vi "BLEwrite_from_file.vi"() -> ()   [LabVIEW 2014]
uses:
  <vilib>/BLE/type_def/address_type.ctl
  <vilib>/BLE/type_def/connection_status_bundle.ctl
panel:
  in  "Control":enum32{"Control Disk", "Diskview from File"}(tab)
  in  "?":bool
  in  "?":bool
  in  "?":bool
  in  "?":bool
  in  "?":bool
  in  "?":bool
  in  "?":bool
  in  "?":bool
  in  "?":bool
  in  "?":bool
  in  "?":bool
  in  "?":bool
  in  "?":bool
  in  "?":bool
  in  "?":bool
  in  "?":bool
  in  "?":bool
  in  "?":bool
  in  "?":bool
  in  "?":bool
  in  "?":bool
  in  "?":bool
  in  "?":bool
  in  "?":bool
  in  "?":bool
  in  "?":bool
  in  "?":bool
  in  "?":bool
  in  "?":bool
  in  "?":bool
  in  "?":bool
  in  "?":bool
  in  "?":bool
  in  "?":bool
  in  "?":bool
  in  "?":bool
  in  "?":bool
  in  "?":bool
  in  "?":bool
  in  "?":bool
  in  "?":bool
  in  "?":bool
  in  "?":bool
  in  "?":bool
  in  "?":bool
  in  "?":bool
  in  "?":bool
  in  "?":bool
  in  "?":bool
  in  "?":bool
  in  "?":bool
  in  "?":bool
  in  "?":bool
  in  "?":bool
  in  "?":bool
  in  "?":bool
  in  "?":bool
  in  "?":bool
  in  "?":bool
  in  "?":bool
  in  "?":bool
  in  "?":bool
  in  "?":bool
  in  "?":bool
  in  "?":bool
  in  "?":bool
  in  "?":bool
  in  "?":bool
  in  "?":bool
  in  "?":bool
  in  "?":bool
  in  "?":bool
  in  "?":bool
  in  "?":bool
  in  "?":bool
  in  "?":bool
  in  "?":bool
  in  "?":bool
  in  "?":bool
  in  "?":bool
  in  "?":bool
  in  "?":bool
  in  "?":bool
  in  "?":bool
  in  "?":bool
  in  "?":bool
  in  "?":bool
  in  "?":bool
  in  "?":bool
  in  "?":bool
  in  "?":bool
  in  "?":bool
  in  "?":bool
  in  "?":bool
  in  "?":bool
  in  "?":bool
  in  "?":bool
  in  "?":bool
  in  "?":bool
  in  "?":bool
  in  "?":bool
  in  "?":bool
  in  "?":bool
  in  "?":bool
  in  "?":bool
  in  "?":bool
  in  "?":bool
  in  "?":bool
  in  "?":bool
  in  "?":bool
  in  "?":bool
  in  "?":bool
  in  "?":bool
  in  "?":bool
  in  "?":bool
  in  "?":bool
  in  "?":bool
  in  "?":bool
  in  "?":bool
  in  "?":bool
  in  "?":bool
  in  "?":bool
  in  "?":bool
  in  "?":bool
  in  "?":bool
  in  "?":bool
  in  "?":bool
  in  "?":bool
  out "Data sent":u8[](array[numeric]) format="%x"
  out "Expander":string
  out "Valve":string
  out "Write to device":bool
  out "Write from file":bool
  out "text":string[](array[string])
  out "Data sent 2":u8[](array[numeric]) format="%x"
  in  "file (use dialog)":path
  out "Expander 2":string
  out "Valve 2":string
  out "element":string
  out "Number of strings":i32
  out "?":bool
  out "?":bool
  out "?":bool
  out "?":bool
  out "?":bool
  out "?":bool
  out "?":bool
  out "?":bool
  out "?":bool
  out "?":bool
  out "?":bool
  out "?":bool
  out "?":bool
  out "?":bool
  out "?":bool
  out "?":bool
  out "?":bool
  out "?":bool
  out "?":bool
  out "?":bool
  out "?":bool
  out "?":bool
  out "?":bool
  out "?":bool
  out "?":bool
  out "?":bool
  out "?":bool
  out "?":bool
  out "?":bool
  out "?":bool
  out "?":bool
  out "?":bool
  out "?":bool
  out "?":bool
  out "?":bool
  out "?":bool
  out "?":bool
  out "?":bool
  out "?":bool
  out "?":bool
  out "?":bool
  out "?":bool
  out "?":bool
  out "?":bool
  out "?":bool
  out "?":bool
  out "?":bool
  out "?":bool
  out "?":bool
  out "?":bool
  out "?":bool
  out "?":bool
  out "?":bool
  out "?":bool
  out "?":bool
  out "?":bool
  out "?":bool
  out "?":bool
  out "?":bool
  out "?":bool
  out "?":bool
  out "?":bool
  out "?":bool
  out "?":bool
  out "?":bool
  out "?":bool
  out "?":bool
  out "?":bool
  out "?":bool
  out "?":bool
  out "?":bool
  out "?":bool
  out "?":bool
  out "?":bool
  out "?":bool
  out "?":bool
  out "?":bool
  out "?":bool
  out "?":bool
  out "?":bool
  out "?":bool
  out "?":bool
  out "?":bool
  out "?":bool
  out "?":bool
  out "?":bool
  out "?":bool
  out "?":bool
  out "?":bool
  out "?":bool
  out "?":bool
  out "?":bool
  out "?":bool
  out "?":bool
  out "?":bool
  out "?":bool
  out "?":bool
  out "?":bool
  out "?":bool
  out "?":bool
  out "?":bool
  out "?":bool
  out "?":bool
  out "?":bool
  out "?":bool
  out "?":bool
  out "?":bool
  out "?":bool
  out "?":bool
  out "?":bool
  out "?":bool
  out "?":bool
  out "?":bool
  out "?":bool
  out "?":bool
  out "?":bool
  out "?":bool
  out "?":bool
  out "?":bool
  out "?":bool
  out "?":bool
  out "?":bool
  out "?":bool
  out "?":bool
  out "?":bool
  out "?":bool
  out "?":bool
  out "?":bool
  in  "Mode Control":bool
  out "Expander Array":bool[](array[boolean])
  out "Expander number":u32
  in  "stop":bool
  out "Discover handles":bool
  out "Handle table":string[][](array[string])
  out "Disconnect":bool
  out "Connection Status":T1={"MAC Address"="", "cnx handle"=0, "cnx flags"=0, "Address Type"=125, "Connection Interval (ms)"=125, "Timeout(ms)"=125, "Latency"=0, "bonding handle"=0} {"Address Type" items=["Public", "Random"]}
  out "Connect to device":bool
  in  "Address Type":T2=1 items=["Public", "Random"]
  in  "MAC Address":string
  in  "COM Bluegiga in":refnum<visa-resource-name>="COM13"
  out "BLED112 Dongle Info":string
  # "Mac Adress: 7C:EC:79:69:6D:AE"
  # "Disk View"
  # "From file"
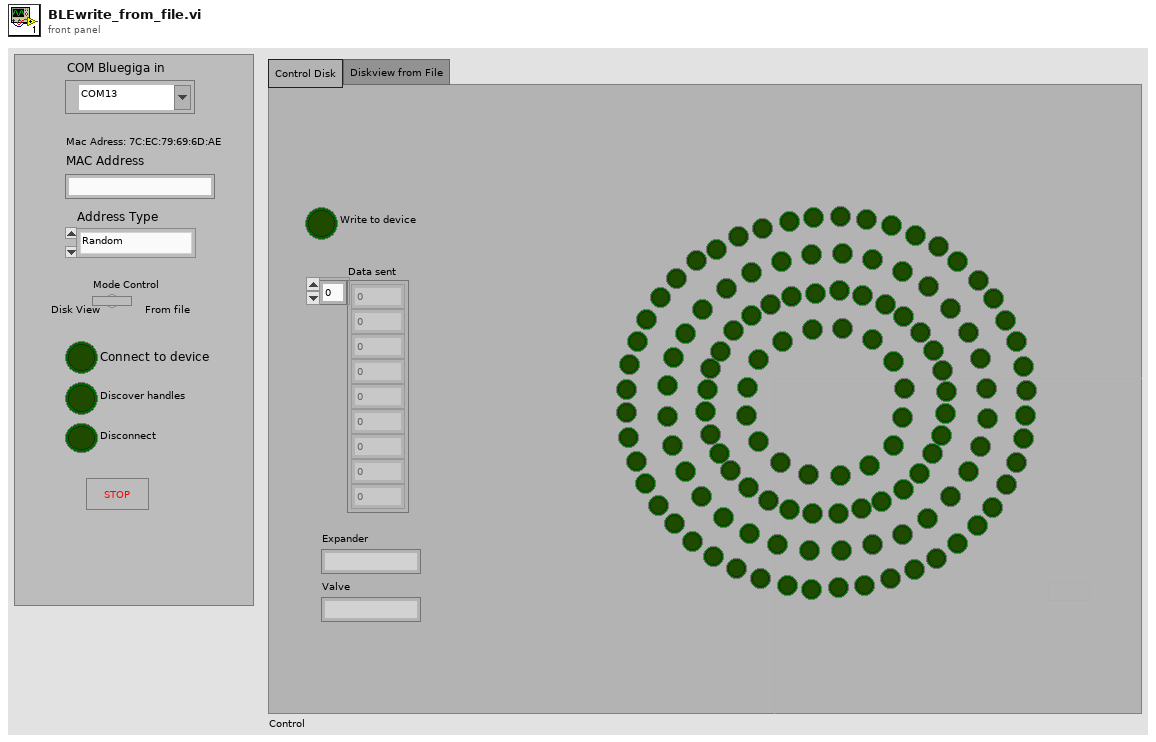
[diagram p1: front panel]
types:
  T1 = typedef "connection_status_bundle.ctl" = cluster{"MAC Address":string, "cnx handle":u8, "cnx flags":u8, "Address Type":T2, "Connection Interval (ms)":u16, "Timeout(ms)":u16, "Latency":u16, "bonding handle":u8}
  T2 = typedef "address_type.ctl" = u8
  T3 = cluster{"[0]":bool, "[1]":bool, "[2]":bool, "[3]":bool, "[4]":bool, "[5]":bool, "[6]":bool, "[7]":bool, "[8]":bool}
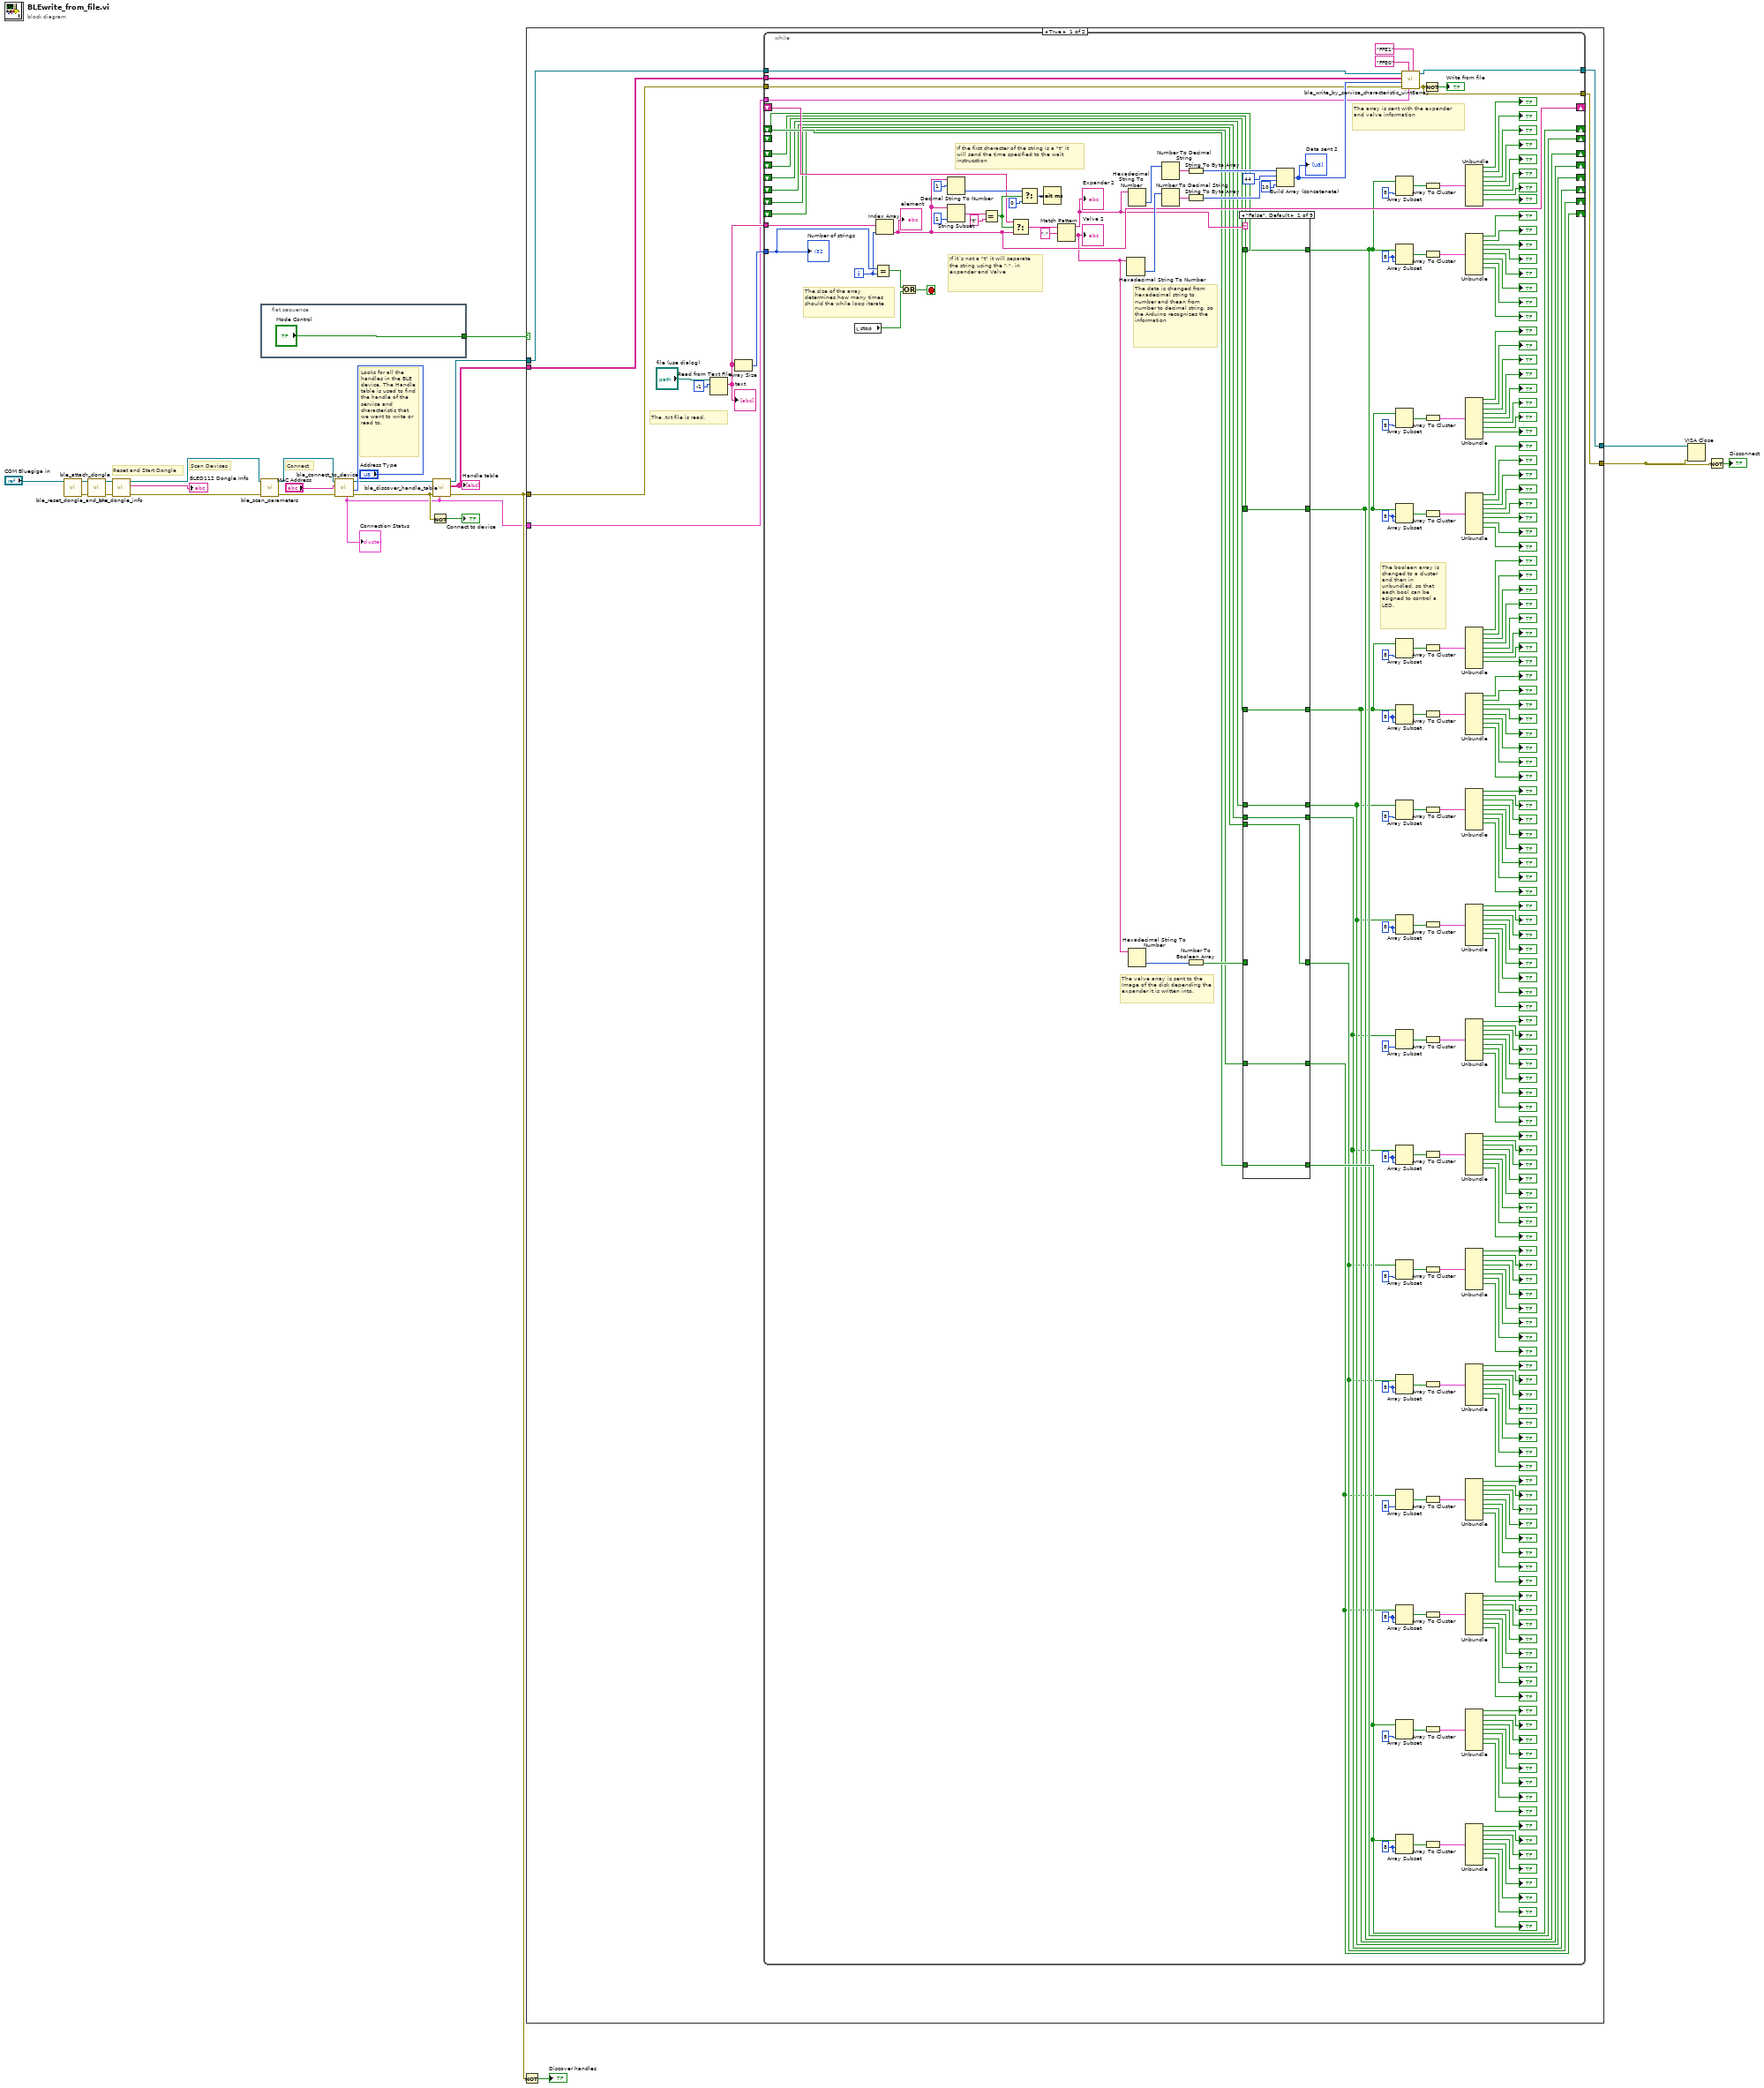
[diagram p0: block diagram]
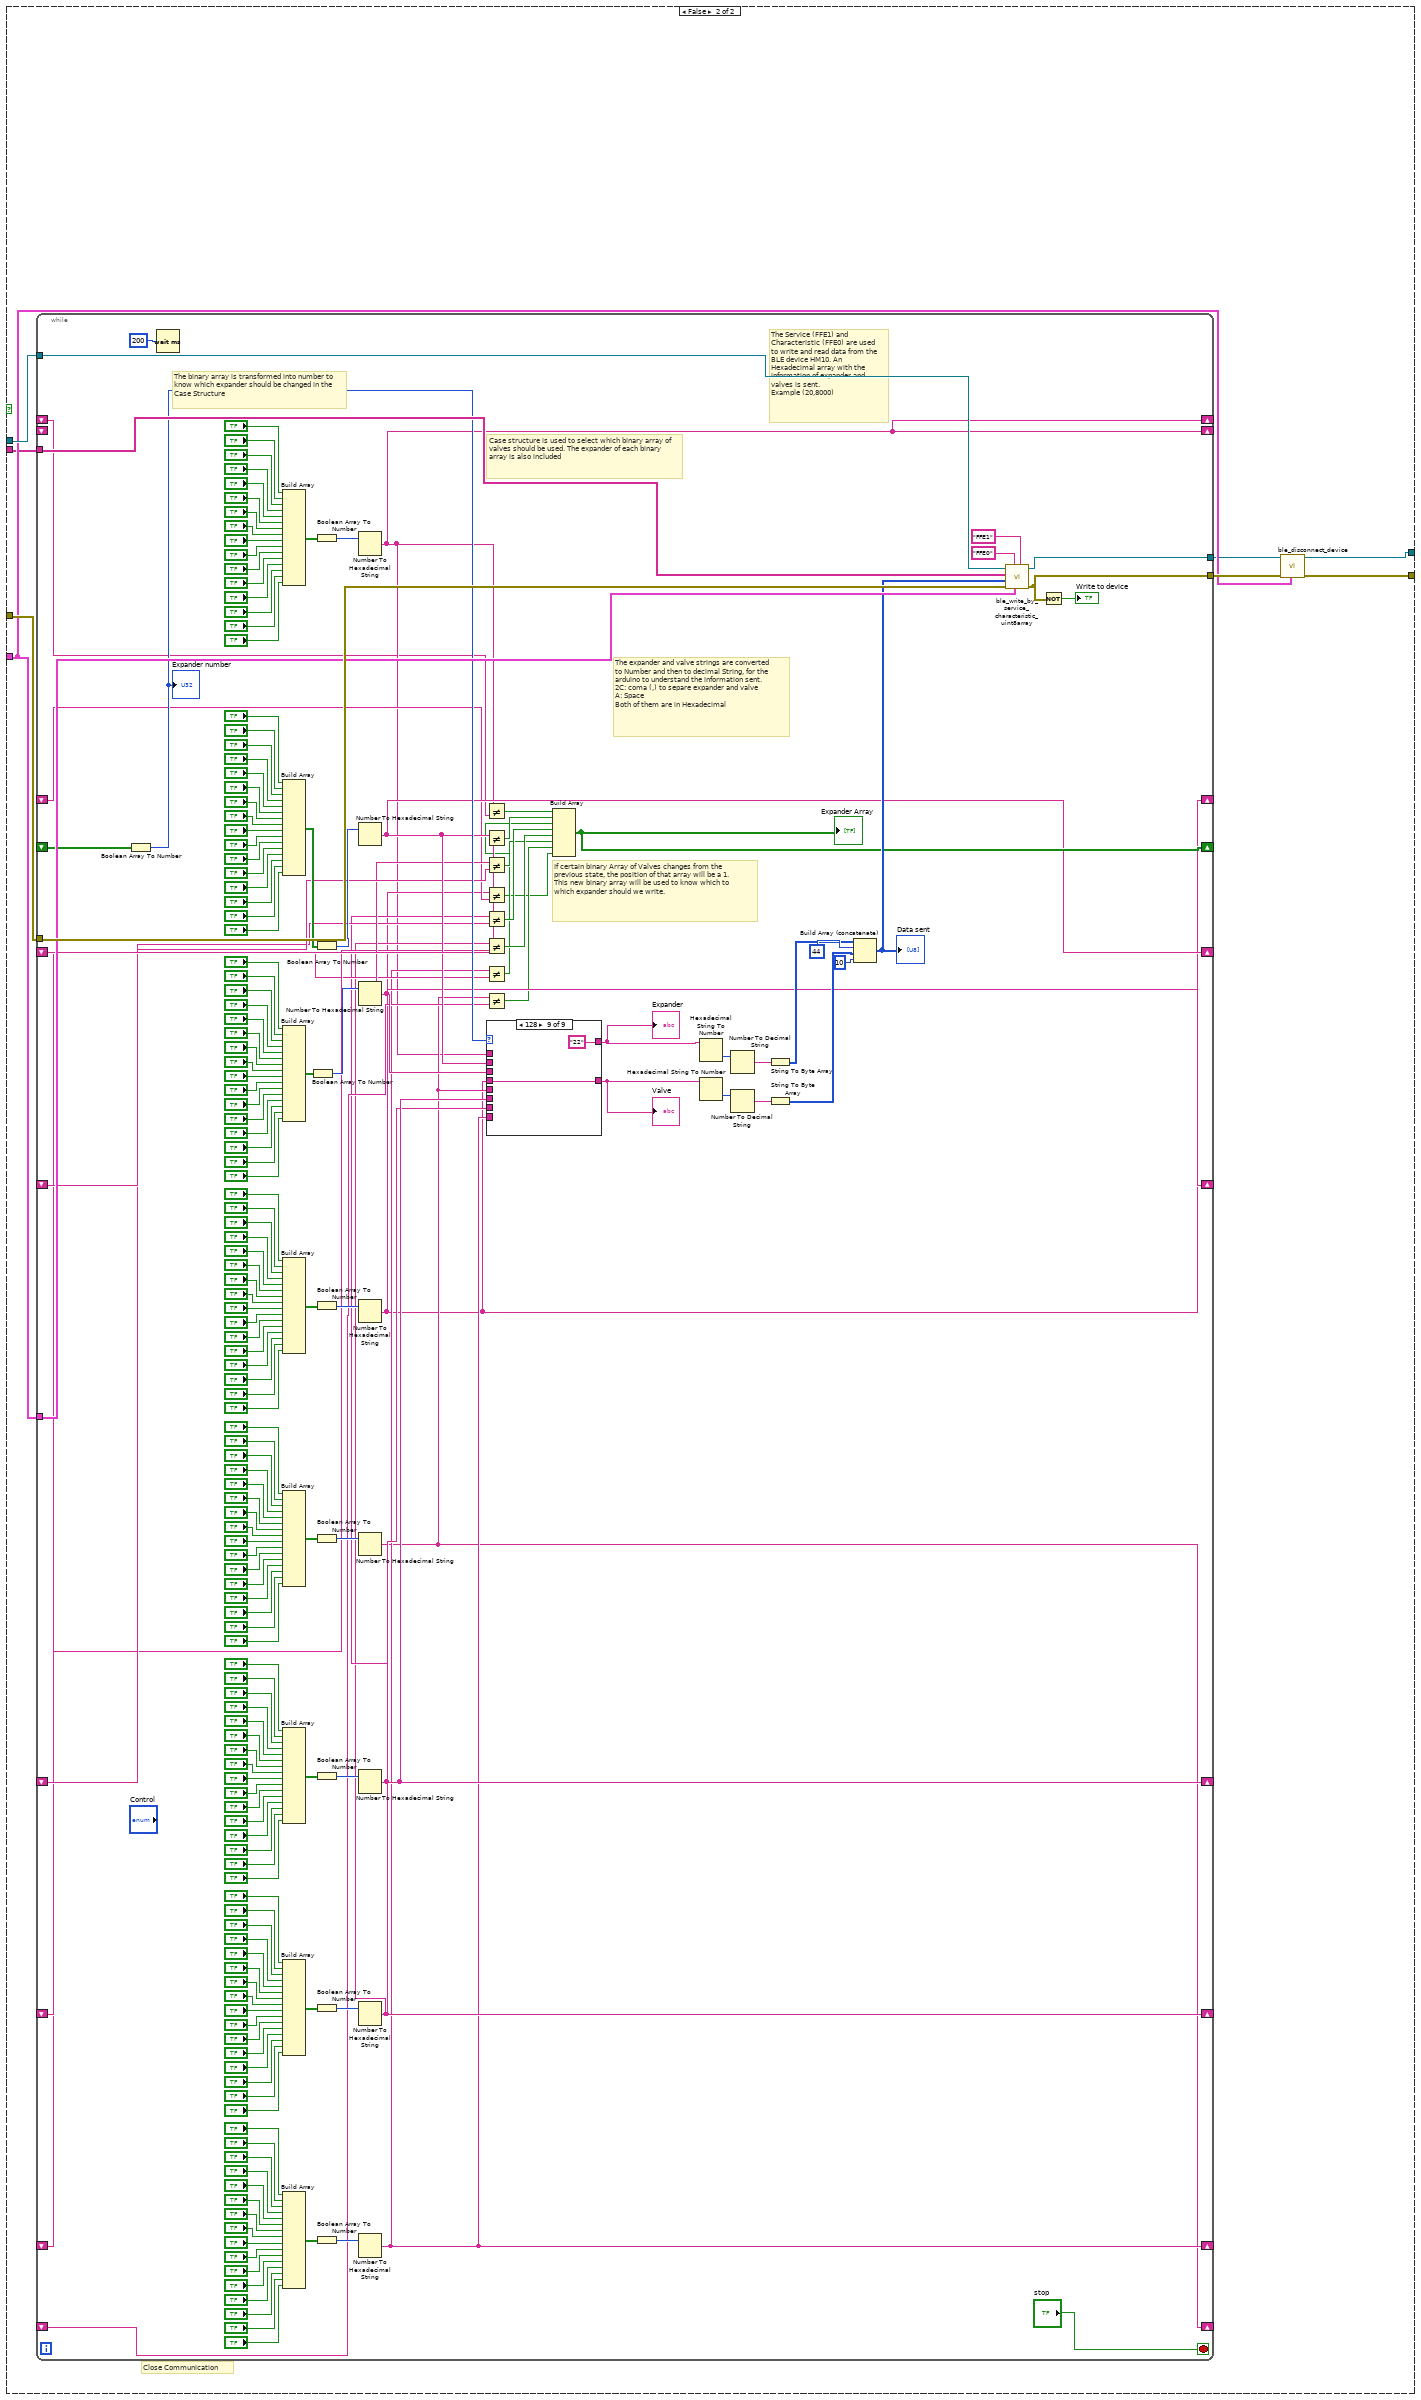
[diagram p10: hidden frame]
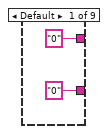
[diagram p11: hidden frame]
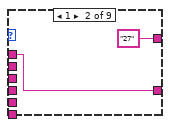
[diagram p12: hidden frame]
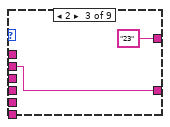
[diagram p13: hidden frame]
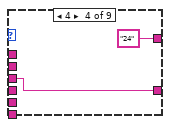
[diagram p14: hidden frame]
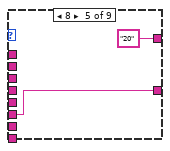
[diagram p15: hidden frame]
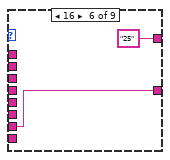
[diagram p16: hidden frame]
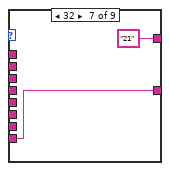
[diagram p17: hidden frame]
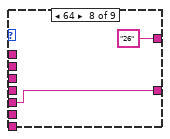
[diagram p18: hidden frame]
diagram:
  # "Reset and Start Dongle"
  # "Scan Devices"
  # "Connect"
  # "Looks for all the handles in the BLE device. The Handle table is used to find the handle of the service and characteristic that we want to write or read to."
  n1 = call <vilib>:"ble_reset_dongle_and_cnx.vi"("COM Bluegiga in"="COM Bluegiga in") -> ("error out"=w19:errorcluster, "COM Bluegiga out"=w17:refnum<visa-resource-name>)  [unwired: 9 in]
  n2 = call <vilib>:"ble_attach_dongle.vi"("error in (no error)"=w19, "COM Bluegiga in"=w17) -> ("error out"=w21:errorcluster, "COM Bluegiga out"=w20:refnum<visa-resource-name>)  [unwired: 8 in]
  n3 = call <vilib>:"ble_dongle_info.vi"("error in (no error)"=w21, "COM Bluegiga in"=w20) -> ("error out"=w22:errorcluster, "info"=→"BLED112 Dongle Info":string, "COM Bluegiga out"=w23:refnum<visa-resource-name>)  [unwired: 7 in]
  n4 = flat-sequence {
    tunnel: ["Mode Control"] -> w1
    frame #0 {
    }
  }
  n5 = call <vilib>:"ble_scan_parameters.vi"("error in (no error)"=w22, "COM Bluegiga in"=w23) -> ("error out"=w13:errorcluster, "COM Bluegiga out"=w14:refnum<visa-resource-name>)  [unwired: 7 in, 1 out]
  n6 = call <vilib>:"ble_connect_to_device.vi"("Address Type"="Address Type", "error in (no error)"=w13, "MAC Address"="MAC Address", "COM Bluegiga in"=w14) -> ("error out"=w7:errorcluster, "COM Bluegiga out"=w8:refnum<visa-resource-name>, "Connection Status"=w3:T1)  [unwired: 5 in]
  "Connection Status" <- w3
  n7 = Not(x=w7) -> (.not. x?=→"Connect to device":bool)
  n8 = call <vilib>:"ble_discover_handle_table.vi"("Connection Status"=w3, "error in (no error)"=w7, "COM Bluegiga in"=w8) -> ("error out"=w4:errorcluster, "Handle table"=w2:string[][], "COM Bluegiga out"=w5:refnum<visa-resource-name>)  [unwired: 6 in]
  "Handle table" <- w2
  n9 = Not(x=w4) -> (.not. x?=→"Discover handles":bool)
  n10 = case shown="True" w1 {
    tunnel: [w27 w347] -> w11
    tunnel: [w26 w346] -> w9
    tunnel: w5 -> [w30 w345]
    tunnel: w4 -> [w29 w344]
    tunnel: w3 -> [w28 w342]
    tunnel: w2 -> [w31 w341]
    frame True {
      # "The .txt file is read."
      n11 = Read from Text File(file (use dialog)="file (use dialog)", count=-1) -> (text=w32:string[])  [unwired: 2 in, 3 out]
      "text" <- w32
      n12 = Array Size(array=w32) -> (size(s)=w33:i32)
      n13 = while {
        tunnel: w33 -> [w267]
        tunnel: w32 -> [w253]
        tunnel: w31 -> [w251]
        tunnel: w30 -> [w250]
        tunnel: w29 -> [w249]
        tunnel: w28 -> [w248]
        tunnel: [w247] -> w27
        tunnel: [w246] -> w26
        shift-right: [w213] -> _
        shift-left: _ -> [w214]
        shift-right: [w54] -> _
        shift-left: _ -> [w53]
        shift-right: [w52] -> _
        shift-left: _ -> [w51]
        shift-right: [w50] -> _
        shift-left: _ -> [w49]
        shift-right: [w48] -> _
        shift-left: _ -> [w47]
        shift-right: [w46] -> _
        shift-left: _ -> [w45]
        shift-right: [w44] -> _
        shift-left: _ -> [w43]
        shift-right: [w42] -> _
        shift-left: _ -> [w41]
        shift-right: [w40] -> _
        shift-left: _ -> [w39]
        i -> [w254]
        stop <- w36 stop-if-true
        w170 = 8 ("length 2")
        w176 = 8 ("length 2")
        w182 = 8 ("length 2")
        w188 = 8 ("length 2")
        w194 = 8 ("length 2")
        w200 = 8 ("length 2")
        w206 = 8 ("length 2")
        w233 = 8 ("length 2")
        # "The boolean array is changed to a cluster and then in unbundled, so that each bool can be asigned to control a LED."
        # "The valve array is sent to the Image of the disk depending the expander it is written into."
        # "The data is changed from hexadecimal string to number and thean from number to decimal string, so the Arduino recognizes the information"
        # "The array is sent with the expander and valve information"
        # "If it´s not a \"t\" it will separate the string using the \",\", in expander and Valve"
        # "If the first character of the string is a \"t\" it will send the time specified to the wait instrucction"
        # "The size of the array determines how many times should the while loop iterate"
        n14 = local read "stop"() -> (w37:bool)
        n15 = Equal?(x=w267, y=w254) -> (x = y?=w38:bool)
        n16 = Index Array(array=w253, index=w254) -> (element=w213:string)
        "element" <- w213
        n17 = Or(x=w38, y=w37) -> (x .or. y?=w36:bool)
        n18 = Decimal String To Number(string=w213, offset=1 ("offset (0)")) -> (number=w240:i32)  [unwired: 1 in, 1 out]
        n19 = String Subset(string=w213, length (rest)=1 ("length (rest)")) -> (substring=w244:string)  [unwired: 1 in]
        n20 = Equal?(x=w244, y="t") -> (x = y?=w241:bool)
        n21 = Select(t=w214, s=w241, f=w213) -> (s? t:f=w242:string)
        n22 = Select(t=w240, s=w241, f=0) -> (s? t:f=w239:i32)
        n23 = Wait (ms)(milliseconds to wait=w239) -> ()  [unwired: 1 out]
        n24 = Match Pattern(string=w242, regular expression=",") -> (before substring=w210:string, after substring=w212:string)  [unwired: 1 in, 2 out]
        "Expander 2" <- w210
        "Valve 2" <- w212
        n25 = Hexadecimal String To Number(string=w212) -> (number=w260:u32)  [unwired: 2 in, 1 out]
        n26 = Hexadecimal String To Number(string=w210) -> (number=w263:u32)  [unwired: 2 in, 1 out]
        n27 = Hexadecimal String To Number(string=w212) -> (number=w211:u32)  [unwired: 2 in, 1 out]
        n28 = Number To Decimal String(number=w263) -> (decimal integer string=w262:string)  [unwired: 1 in]
        n29 = Number To Decimal String(number=w260) -> (decimal integer string=w259:string)  [unwired: 1 in]
        n30 = String To Byte Array(string=w262) -> (unsigned byte array=w257:u8[])
        n31 = String To Byte Array(string=w259) -> (unsigned byte array=w258:u8[])
        n32 = Number To Boolean Array(number=w211) -> (Boolean array=w55:bool[])
        n33 = case shown="\"False\", Default" w210 {
          tunnel: [w275 w283 w290 w299 w307 w315 w323 w331 w339] -> w54
          tunnel: w55 -> [_ w283 w291 w297 w304 w311 w318 w325 w332]
          tunnel: [w274 w282 w291 w298 w306 w314 w322 w330 w338] -> w52
          tunnel: w53 -> [w275 _ w290 w299 w307 w315 w323 w331 w339]
          tunnel: w51 -> [w274 w282 _ w298 w306 w314 w322 w330 w338]
          tunnel: [w273 w281 w289 w297 w305 w313 w321 w329 w337] -> w50
          tunnel: w49 -> [w273 w281 w289 _ w305 w313 w321 w329 w337]
          tunnel: [w272 w280 w288 w296 w304 w312 w320 w328 w336] -> w48
          tunnel: w47 -> [w272 w280 w288 w296 _ w312 w320 w328 w336]
          tunnel: [w271 w279 w287 w295 w303 w311 w319 w327 w335] -> w46
          tunnel: w45 -> [w271 w279 w287 w295 w303 _ w319 w327 w335]
          tunnel: [w270 w278 w286 w294 w302 w310 w318 w326 w334] -> w44
          tunnel: w43 -> [w270 w278 w286 w294 w302 w310 _ w326 w334]
          tunnel: [w269 w277 w285 w293 w301 w309 w317 w325 w333] -> w42
          tunnel: w41 -> [w269 w277 w285 w293 w301 w309 w317 _ w333]
          tunnel: [w268 w276 w284 w292 w300 w308 w316 w324 w332] -> w40
          tunnel: w39 -> [w268 w276 w284 w292 w300 w308 w316 w324 _]
          frame "False", Default {
          }
          frame "27" {
          }
          frame "23" {
          }
          frame "24" {
          }
          frame "22" {
          }
          frame "26" {
          }
          frame "20" {
          }
          frame "25" {
          }
          frame "21" {
          }
        }
        n34 = Build Array (concatenate)(w257, u8 44 ("number"), w258, u8 10 ("number")) -> (w255:u8[])
        "Data sent 2" <- w255
        n35 = Array Subset(array=w52, length=8 ("length 2")) -> (w205:bool[])  [unwired: 1 in]
        n36 = Array Subset(array=w52, index=w206, length=w206) -> (w204:bool[])
        n37 = Array Subset(array=w50, length=8 ("length 2")) -> (w199:bool[])  [unwired: 1 in]
        n38 = Array Subset(array=w50, index=w200, length=w200) -> (w198:bool[])
        n39 = Array Subset(array=w48, length=8 ("length 2")) -> (w193:bool[])  [unwired: 1 in]
        n40 = Array Subset(array=w48, index=w194, length=w194) -> (w192:bool[])
        n41 = Array Subset(array=w46, length=8 ("length 2")) -> (w187:bool[])  [unwired: 1 in]
        n42 = Array Subset(array=w46, index=w188, length=w188) -> (w186:bool[])
        n43 = Array Subset(array=w44, length=8 ("length 2")) -> (w181:bool[])  [unwired: 1 in]
        n44 = Array Subset(array=w44, index=w182, length=w182) -> (w180:bool[])
        n45 = Array Subset(array=w42, length=8 ("length 2")) -> (w175:bool[])  [unwired: 1 in]
        n46 = Array Subset(array=w42, index=w176, length=w176) -> (w174:bool[])
        n47 = Array Subset(array=w40, length=8 ("length 2")) -> (w169:bool[])  [unwired: 1 in]
        n48 = Array Subset(array=w40, index=w170, length=w170) -> (w168:bool[])
        n49 = Array Subset(array=w54, length=8 ("length 2")) -> (w232:bool[])  [unwired: 1 in]
        n50 = Array Subset(array=w54, index=w233, length=w233) -> (w231:bool[])
        n51 = call <vilib>:"ble_write_by_service_characteristic_uint8array.vi"("Characteristic UUID"="FFE1", "Connection Status"=w248, "Service UUID"="FFE0", "error in (no error)"=w249, "data"=w255, "Handle table"=w251, "COM Bluegiga in"=w250) -> ("error out"=w246:errorcluster, "COM Bluegiga out"=w247:refnum<visa-resource-name>)  [unwired: 3 in]
        n52 = Not(x=w246) -> (.not. x?=→"Write from file":bool)
        n53 = Array To Cluster(array=w205) -> (cluster=w209:T3)
        n54 = Array To Cluster(array=w204) -> (cluster=w208:T3)
        n55 = Array To Cluster(array=w199) -> (cluster=w203:T3)
        n56 = Array To Cluster(array=w198) -> (cluster=w202:T3)
        n57 = Array To Cluster(array=w193) -> (cluster=w197:T3)
        n58 = Array To Cluster(array=w192) -> (cluster=w196:T3)
        n59 = Array To Cluster(array=w187) -> (cluster=w191:T3)
        n60 = Array To Cluster(array=w186) -> (cluster=w190:T3)
        n61 = Array To Cluster(array=w181) -> (cluster=w185:T3)
        n62 = Array To Cluster(array=w180) -> (cluster=w184:T3)
        n63 = Array To Cluster(array=w175) -> (cluster=w179:T3)
        n64 = Array To Cluster(array=w174) -> (cluster=w178:T3)
        n65 = Array To Cluster(array=w169) -> (cluster=w173:T3)
        n66 = Array To Cluster(array=w168) -> (cluster=w172:T3)
        n67 = Array To Cluster(array=w232) -> (cluster=w236:T3)
        n68 = Array To Cluster(array=w231) -> (cluster=w235:T3)
        n69 = Unbundle(w209) -> ("[0]"=→"?":bool, "[1]"=→"?":bool, "[2]"=→"?":bool, "[3]"=→"?":bool, "[4]"=→"?":bool, "[5]"=→"?":bool, "[6]"=→"?":bool, "[7]"=→"?":bool)  [unwired: 1 out]
        n70 = Unbundle(w208) -> ("[0]"=→"?":bool, "[1]"=→"?":bool, "[2]"=→"?":bool, "[3]"=→"?":bool, "[4]"=→"?":bool, "[5]"=→"?":bool, "[6]"=→"?":bool, "[7]"=→"?":bool)  [unwired: 1 out]
        n71 = Unbundle(w203) -> ("[0]"=→"?":bool, "[1]"=→"?":bool, "[2]"=→"?":bool, "[3]"=→"?":bool, "[4]"=→"?":bool, "[5]"=→"?":bool, "[6]"=→"?":bool, "[7]"=→"?":bool)  [unwired: 1 out]
        n72 = Unbundle(w202) -> ("[0]"=→"?":bool, "[1]"=→"?":bool, "[2]"=→"?":bool, "[3]"=→"?":bool, "[4]"=→"?":bool, "[5]"=→"?":bool, "[6]"=→"?":bool, "[7]"=→"?":bool)  [unwired: 1 out]
        n73 = Unbundle(w197) -> ("[0]"=→"?":bool, "[1]"=→"?":bool, "[2]"=→"?":bool, "[3]"=→"?":bool, "[4]"=→"?":bool, "[5]"=→"?":bool, "[6]"=→"?":bool, "[7]"=→"?":bool)  [unwired: 1 out]
        n74 = Unbundle(w196) -> ("[0]"=→"?":bool, "[1]"=→"?":bool, "[2]"=→"?":bool, "[3]"=→"?":bool, "[4]"=→"?":bool, "[5]"=→"?":bool, "[6]"=→"?":bool, "[7]"=→"?":bool)  [unwired: 1 out]
        n75 = Unbundle(w191) -> ("[0]"=→"?":bool, "[1]"=→"?":bool, "[2]"=→"?":bool, "[3]"=→"?":bool, "[4]"=→"?":bool, "[5]"=→"?":bool, "[6]"=→"?":bool, "[7]"=→"?":bool)  [unwired: 1 out]
        n76 = Unbundle(w190) -> ("[0]"=→"?":bool, "[1]"=→"?":bool, "[2]"=→"?":bool, "[3]"=→"?":bool, "[4]"=→"?":bool, "[5]"=→"?":bool, "[6]"=→"?":bool, "[7]"=→"?":bool)  [unwired: 1 out]
        n77 = Unbundle(w185) -> ("[0]"=→"?":bool, "[1]"=→"?":bool, "[2]"=→"?":bool, "[3]"=→"?":bool, "[4]"=→"?":bool, "[5]"=→"?":bool, "[6]"=→"?":bool, "[7]"=→"?":bool)  [unwired: 1 out]
        n78 = Unbundle(w184) -> ("[0]"=→"?":bool, "[1]"=→"?":bool, "[2]"=→"?":bool, "[3]"=→"?":bool, "[4]"=→"?":bool, "[5]"=→"?":bool, "[6]"=→"?":bool, "[7]"=→"?":bool)  [unwired: 1 out]
        n79 = Unbundle(w179) -> ("[0]"=→"?":bool, "[1]"=→"?":bool, "[2]"=→"?":bool, "[3]"=→"?":bool, "[4]"=→"?":bool, "[5]"=→"?":bool, "[6]"=→"?":bool, "[7]"=→"?":bool)  [unwired: 1 out]
        n80 = Unbundle(w178) -> ("[0]"=→"?":bool, "[1]"=→"?":bool, "[2]"=→"?":bool, "[3]"=→"?":bool, "[4]"=→"?":bool, "[5]"=→"?":bool, "[6]"=→"?":bool, "[7]"=→"?":bool)  [unwired: 1 out]
        n81 = Unbundle(w173) -> ("[0]"=→"?":bool, "[1]"=→"?":bool, "[2]"=→"?":bool, "[3]"=→"?":bool, "[4]"=→"?":bool, "[5]"=→"?":bool, "[6]"=→"?":bool, "[7]"=→"?":bool)  [unwired: 1 out]
        n82 = Unbundle(w172) -> ("[0]"=→"?":bool, "[1]"=→"?":bool, "[2]"=→"?":bool, "[3]"=→"?":bool, "[4]"=→"?":bool, "[5]"=→"?":bool, "[6]"=→"?":bool, "[7]"=→"?":bool)  [unwired: 1 out]
        n83 = Unbundle(w236) -> ("[0]"=→"?":bool, "[1]"=→"?":bool, "[2]"=→"?":bool, "[3]"=→"?":bool, "[4]"=→"?":bool, "[5]"=→"?":bool, "[6]"=→"?":bool, "[7]"=→"?":bool)  [unwired: 1 out]
        n84 = Unbundle(w235) -> ("[0]"=→"?":bool, "[1]"=→"?":bool, "[2]"=→"?":bool, "[3]"=→"?":bool, "[4]"=→"?":bool, "[5]"=→"?":bool, "[6]"=→"?":bool, "[7]"=→"?":bool)  [unwired: 1 out]
        "Number of strings" <- w267
      }
    }
    frame False {
      # "Close Communication"
      n85 = while {
        tunnel: w345 -> [w536]
        tunnel: w344 -> [w534]
        tunnel: [w531] -> w343
        tunnel: [w533] -> w340
        tunnel: w342 -> [w532]
        tunnel: w341 -> [w535]
        shift-right: [w350] -> _
        shift-left: _ -> [_]
        shift-right: [w477] -> _
        shift-left: _ -> [w478]
        shift-right: [w483] -> _
        shift-left: _ -> [w482]
        shift-right: [w456] -> _
        shift-left: _ -> [w458]
        shift-right: [w356] -> _
        shift-left: _ -> [w366]
        shift-right: [w355] -> _
        shift-left: _ -> [w365]
        shift-right: [w354] -> _
        shift-left: _ -> [w364]
        shift-right: [w353] -> _
        shift-left: _ -> [w363]
        shift-right: [w352] -> _
        shift-left: _ -> [w362]
        shift-right: [w350] -> _
        shift-left: _ -> [w349]
        stop <- "stop" stop-if-true
        # "The Service (FFE1) and Characteristic (FFE0) are used to write and read data from the BLE device HM10. An Hexadecimal array with the information of expander and valves is sent.\nExample (20,8000)"
        # "The expander and valve strings are converted to Number and then to decimal String, for the arduino to understand the information sent. \n2C: coma (,) to separe expander and valve\nA: Space\nBoth of them are in Hexadecimal"
        # "Case structure is used to select which binary array of valves should be used. The expander of each binary array is also included"
        # "The binary array is transformed into number to know which expander should be changed in the Case Structure"
        # "If certain binary Array of Valves changes from the previous state, the position of that array will be a 1. This new binary array will be used to know which to which expander should we write."
        n86 = Boolean Array To Number(Boolean array=w482) -> (number=w481:u32)
        "Expander number" <- w481
        n87 = Wait (ms)(milliseconds to wait=u32 200) -> ()  [unwired: 1 out]
        n88 = Build Array("?", "?", "?", "?", "?", "?", "?", "?", "?", "?", "?", "?", "?", "?", "?", "?") -> (w505:bool[])
        n89 = Build Array("?", "?", "?", "?", "?", "?", "?", "?", "?", "?", "?", "?", "?", "?", "?", "?") -> (w503:bool[])
        n90 = Build Array("?", "?", "?", "?", "?", "?", "?", "?", "?", "?", "?", "?", "?", "?", "?", "?") -> (w476:bool[])
        n91 = Build Array("?", "?", "?", "?", "?", "?", "?", "?", "?", "?", "?", "?", "?", "?", "?", "?") -> (w446:bool[])
        n92 = Build Array("?", "?", "?", "?", "?", "?", "?", "?", "?", "?", "?", "?", "?", "?", "?", "?") -> (w448:bool[])
        n93 = Build Array("?", "?", "?", "?", "?", "?", "?", "?", "?", "?", "?", "?", "?", "?", "?", "?") -> (w454:bool[])
        n94 = Build Array("?", "?", "?", "?", "?", "?", "?", "?", "?", "?", "?", "?", "?", "?", "?", "?") -> (w452:bool[])
        n95 = Build Array("?", "?", "?", "?", "?", "?", "?", "?", "?", "?", "?", "?", "?", "?", "?", "?") -> (w450:bool[])
        n96 = Boolean Array To Number(Boolean array=w476) -> (number=w475:u32)
        n97 = Boolean Array To Number(Boolean array=w505) -> (number=w504:u32)
        n98 = Boolean Array To Number(Boolean array=w503) -> (number=w502:u32)
        n99 = Boolean Array To Number(Boolean array=w446) -> (number=w447:u32)
        n100 = Boolean Array To Number(Boolean array=w448) -> (number=w449:u32)
        n101 = Boolean Array To Number(Boolean array=w454) -> (number=w455:u32)
        n102 = Boolean Array To Number(Boolean array=w452) -> (number=w453:u32)
        n103 = Boolean Array To Number(Boolean array=w450) -> (number=w451:u32)
        n104 = Number To Hexadecimal String(2:w504) -> (0:w350:string)  [unwired: 1 in]
        n105 = Number To Hexadecimal String(2:w502) -> (0:w477:string)  [unwired: 1 in]
        n106 = Number To Hexadecimal String(2:w475) -> (0:w456:string)  [unwired: 1 in]
        n107 = Number To Hexadecimal String(2:w447) -> (0:w352:string)  [unwired: 1 in]
        n108 = Number To Hexadecimal String(2:w449) -> (0:w353:string)  [unwired: 1 in]
        n109 = Number To Hexadecimal String(2:w455) -> (0:w356:string)  [unwired: 1 in]
        n110 = Number To Hexadecimal String(2:w453) -> (0:w355:string)  [unwired: 1 in]
        n111 = Number To Hexadecimal String(2:w451) -> (0:w354:string)  [unwired: 1 in]
        n112 = Not Equal?(x=w350, y=w349) -> (x != y?=w485:bool)
        n113 = Not Equal?(x=w477, y=w478) -> (x != y?=w484:bool)
        n114 = Not Equal?(x=w456, y=w458) -> (x != y?=w457:bool)
        n115 = Not Equal?(x=w356, y=w366) -> (x != y?=w361:bool)
        n116 = Not Equal?(x=w355, y=w365) -> (x != y?=w360:bool)
        n117 = Not Equal?(x=w354, y=w364) -> (x != y?=w359:bool)
        n118 = Not Equal?(x=w353, y=w363) -> (x != y?=w358:bool)
        n119 = Not Equal?(x=w352, y=w362) -> (x != y?=w357:bool)
        n120 = case shown="128" w481 {
          tunnel: ["0" "27" "23" "24" "20" "25" "21" "26" "22"] -> w480
          tunnel: ["0" w543 w545 w547 w549 w551 w553 w555 w557] -> w479
          tunnel: w350 -> [_ w543 _ _ _ _ _ _ _]
          tunnel: w477 -> [_ _ w545 _ _ _ _ _ _]
          tunnel: w456 -> [_ _ _ w547 _ _ _ _ _]
          tunnel: w356 -> [_ _ _ _ w549 _ _ _ _]
          tunnel: w355 -> [_ _ _ _ _ w551 _ _ _]
          tunnel: w354 -> [_ _ _ _ _ _ w553 _ _]
          tunnel: w353 -> [_ _ _ _ _ _ _ w555 _]
          tunnel: w352 -> [_ _ _ _ _ _ _ _ w557]
          frame Default {
          }
          frame 1 {
          }
          frame 2 {
          }
          frame 4 {
          }
          frame 8 {
          }
          frame 16 {
          }
          frame 32 {
          }
          frame 64 {
          }
          frame 128 {
          }
        }
        "Expander" <- w480
        "Valve" <- w479
        n121 = Build Array(w485, w484, w457, w361, w360, w359, w358, w357) -> (w483:bool[])
        "Expander Array" <- w483
        n122 = Hexadecimal String To Number(string=w480) -> (number=w530:u32)  [unwired: 2 in, 1 out]
        n123 = Hexadecimal String To Number(string=w479) -> (number=w527:u32)  [unwired: 2 in, 1 out]
        n124 = Number To Decimal String(number=w530) -> (decimal integer string=w529:string)  [unwired: 1 in]
        n125 = Number To Decimal String(number=w527) -> (decimal integer string=w526:string)  [unwired: 1 in]
        n126 = String To Byte Array(string=w529) -> (unsigned byte array=w524:u8[])
        n127 = String To Byte Array(string=w526) -> (unsigned byte array=w525:u8[])
        n128 = Build Array (concatenate)(w524, u8 44 ("number"), w525, u8 10 ("number")) -> (w522:u8[])
        "Data sent" <- w522
        n129 = call <vilib>:"ble_write_by_service_characteristic_uint8array.vi"("Characteristic UUID"="FFE1", "Connection Status"=w532, "Service UUID"="FFE0", "error in (no error)"=w534, "data"=w522, "Handle table"=w535, "COM Bluegiga in"=w536) -> ("error out"=w531:errorcluster, "COM Bluegiga out"=w533:refnum<visa-resource-name>)  [unwired: 3 in]
        n130 = Not(x=w531) -> (.not. x?=→"Write to device":bool)
      }
      n131 = call <vilib>:"ble_disconnect_device.vi"("Connection Status"=w342, "error in (no error)"=w343, "COM Bluegiga in"=w340) -> ("error out"=w346:errorcluster, "COM Bluegiga out"=w347:refnum<visa-resource-name>)  [unwired: 7 in]
    }
  }
  n132 = VISA Close(VISA resource name=w11, error in (no error)=w9) -> ()  [unwired: 1 out]
  n133 = Not(x=w9) -> (.not. x?=→"Disconnect":bool)
